vi "Sheet Names.vi"(10 "Excel._Worksheet":refnum<k7>, 11 "Worksheets":refnum<k7>) -> (2 "Sheet Name":string[](array[string]), 3 "Excel._Worksheet":refnum<k7>)   [LabVIEW 2017]
panel:
  in  "Error In":errorcluster
  out "error out":errorcluster
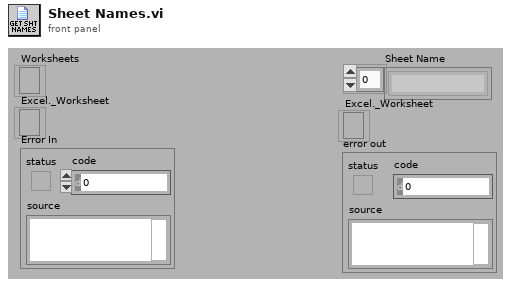
[diagram p1: front panel]
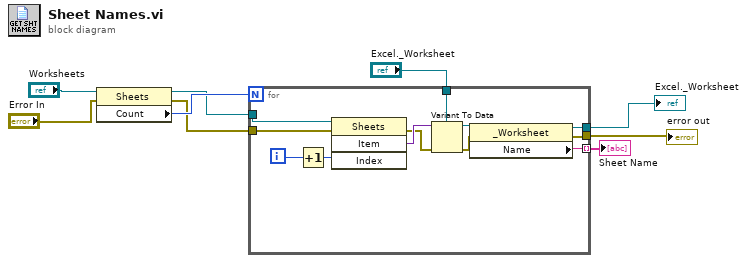
[diagram p0: block diagram]
diagram:
  n1 = property class="Sheets"(reference="Worksheets", error in="Error In") -> (reference out=w7:refnum<k7>, error out=w3:errorcluster, "Count"=w8:i32)
  n2 = for {
    N: w8 -> [_]
    tunnel: w7 -> [w21]
    tunnel: "Excel._Worksheet" -> [w17]
    tunnel: [w15] -> w5 mode=indexing
    tunnel: [w14] -> w4
    tunnel: w3 -> [w13]
    tunnel: [w10] -> w2
    i -> [w20]
    n3 = Increment(x=w20) -> (x+1=w19:i32)
    n4 = invoke class="Sheets" method="Item"(reference=w21, error in=w13, "Index"=w19) -> (error out=w12:errorcluster, "Item"=w18:variant)  [unwired: 1 in, 2 out]
    n5 = Variant To Data(error in=w12, type=w17, Variant=w18) -> (data=w16:refnum<k7>, error out=w11:errorcluster)
    n6 = property class="_Worksheet"(reference=w16, error in=w11) -> (reference out=w14:refnum<k7>, error out=w10:errorcluster, "Name"=w15:string)
  }
  "Sheet Name" <- w5
  "Excel._Worksheet" <- w4
  "error out" <- w2
